vi "G4BaseTemplate_Simple_5x6x5_WriteAttribute.vi"(0 "reference in":refnum<class "G4BaseTemplate_Simple_5x6x5.lvclass">, 11 "error in (no error)":errorcluster) -> (4 "reference out":refnum<class "G4BaseTemplate_Simple_5x6x5.lvclass">, 15 "error out":errorcluster)   [LabVIEW 2014]
uses:
  <resource>/Framework/Providers/Open_GDS/ClassProviders/Provider_EndevoGOOP400/Templates/G4BaseTemplate_Simple_5x6x5/G4BaseTemplate_Simple_5x6x5.lvclass
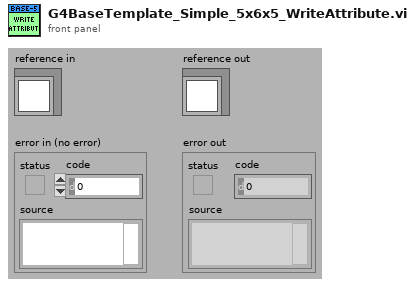
[diagram p1: front panel]
types:
  T1 = typedef "G4BaseTemplate_Simple_5x6x5.lvclass/ObjectAttributes.ctl" = cluster{"Attribute1":dbl}
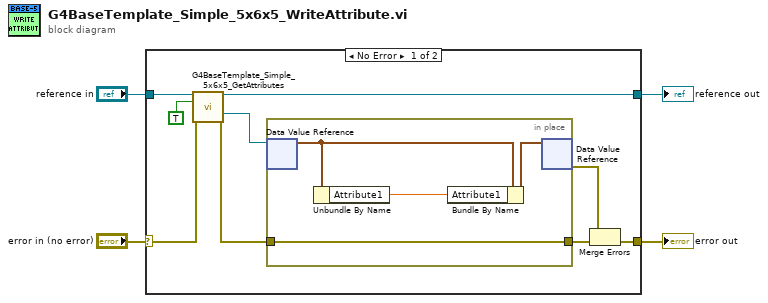
[diagram p0: block diagram]
diagram:
  n1 = case shown="No Error" "error in (no error)" {
    selector: "error in (no error)" -> [w8 w19]
    tunnel: [w12 w19] -> w3
    tunnel: [w10 w18] -> w1
    tunnel: "reference in" -> [w11 w18]
    frame No Error {
      n2 = call <resource>:"G4BaseTemplate_Simple_5x6x5_GetAttributes.vi"("reference in"=w11, "OnlyGetDvrReference(False)"=TRUE, "error in (no error)"=w8) -> ("reference out"=w10:refnum<class "G4BaseTemplate_Simple_5x6x5.lvclass">, "DataRef"=w9:refnum<data-value>, "error out"=w7:errorcluster)  [unwired: 9 in, 1 out]
      n3 = in-place {
        in-place-border: w7 -> [w16]
        in-place-border: [w16] -> w6
        n4 = in-place-dvr #1(w9) -> (w15:T1)  [unwired: 1 out]
        n5 = Unbundle By Name(w15) -> ("Attribute1"=w14:dbl)
        n6 = Bundle By Name(cluster=w15, "Attribute1"=w14) -> (w17:T1)
        n7 = in-place-dvr #1(w17) -> (w13:errorcluster)  [unwired: 1 out]
      }
      n8 = Merge Errors(w13, w6) -> (w12:errorcluster)
    }
    frame Error {
    }
  }
  "error out" <- w3
  "reference out" <- w1
